vi "Get straight position.vi"   [LabVIEW 2016, in "Test2.lvrbt"]
uses:
  Test2.lvrbt
  <vilib>/NXT/Block Support/NXT_InputPort.ctl
  <vilib>/NXT/Hardware/Plugins/Tetrix DC Motor/TetrixDCMotorAddress.ctl
  <vilib>/NXT/Dual Mode Library/Sensors/Light_On.vi
  <vilib>/NXT/NXTIO Xnodes/NXTIONodeSubVIs/TETRIX IO Move DC Motors.vi
  <vilib>/NXT/Dual Mode Library/Waits/Wait_Num(msec).vi
  <vilib>/NXT/NXTIO Xnodes/NXTIONodeSubVIs/TETRIX IO Stop DC Motors.vi
  <vilib>/NXT/Subs/LVHSConnector.ctl
  <vilib>/NXT/NXTIO Xnodes/AddressXNode/NXTIOAddress.xnode
  <vilib>/NXT/NXTIO Xnodes/NXTIOXNode/NXTIO.xnode
  <vilib>/NXT/LegoClasses/BrickReference/BrickReference.lvclass
types:
  T1 = typedef "NXT_InputPort.ctl" = u32
  T2 = typedef "TetrixDCMotorAddress.ctl" = i32
  T3 = typedef "LVHSConnector.ctl" = refnum<class "BrickReference.lvclass">
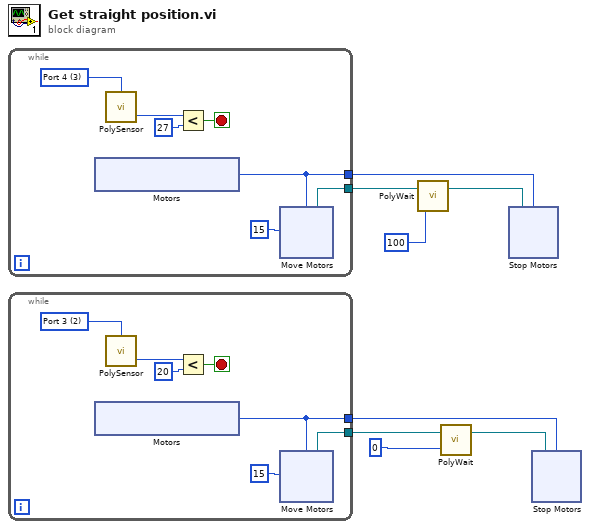
[diagram p0: block diagram]
diagram:
  n1 = while {
    tunnel: [w11] -> w3
    tunnel: [w10] -> w8
    stop <- w12 stop-if-true
    w14 = T1 3 items=["Port 1", "Port 2", "Port 3", "Port 4"] ("Port (Port 3)")
    n2 = xnode "Motors"() -> ("Motor"=w10:T2)
    n3 = call-poly <vilib>:"PolySensor.vi"("Port (Port 3)"=w14) -> ("Scaled Value"=w13:i16)  [unwired: 2 in, 1 out]
    n4 = Less?(x=w13, y=i16 27) -> (x < y?=w12:bool)
    n5 = xnode "Move Motors"("Power/Speed 1"=i8 15, "Motors"=w10) -> ("NXT/EV3"=w11:T3)  [unwired: 1 in]
  }
  n6 = while {
    tunnel: [w26] -> w5
    tunnel: [w25] -> w7
    stop <- w27 stop-if-true
    w29 = T1 2 items=["Port 1", "Port 2", "Port 3", "Port 4"] ("Port (Port 3)")
    n7 = xnode "Motors"() -> ("Motor"=w25:T2)
    n8 = call-poly <vilib>:"PolySensor.vi"("Port (Port 3)"=w29) -> ("Scaled Value"=w28:i16)  [unwired: 2 in, 1 out]
    n9 = Less?(x=w28, y=i16 20) -> (x < y?=w27:bool)
    n10 = xnode "Move Motors"("Power/Speed 1"=i8 15, "Motors"=w25) -> ("NXT/EV3"=w26:T3)  [unwired: 1 in]
  }
  n11 = call-poly <vilib>:"PolyWait.vi"("Time (100 msec)"=u32 100, "NXT/EV3"=w3) -> ("NXT/EV3"=w2:T3)  [unwired: 2 in]
  n12 = call-poly <vilib>:"PolyWait.vi"("Time (100 msec)"=u32 0, "NXT/EV3"=w5) -> ("NXT/EV3"=w4:T3)  [unwired: 2 in]
  n13 = xnode "Stop Motors"("Motors"=w8, "NXT/EV3"=w2) -> ()  [unwired: 1 out]
  n14 = xnode "Stop Motors"("Motors"=w7, "NXT/EV3"=w4) -> ()  [unwired: 1 out]
